vi "Vision Processor.vi"(5 "error in":errorcluster, 7 "Image In":T1) -> (0 "error out":errorcluster, 3 "Image Out":T1(plugin-control))   [LabVIEW 2013]
uses:
  <vilib>/vision/Image Controls.llb/IMAQ Image.ctl
  <vilib>/vision/NI_Vision_Development_Module.lvlib
panel:
  out "Cam":T1(plugin-control)
  # "0  center of mass x\n1  center of mass y\n2  first pixel x\n3  first pixel y\n4  bounding rect left\n5  bounding rect top\n6  bounding rect right\n7  bounding rect bottom\n8 max feret diameter start x\n9  max feret diameter start y\n10 max feret diameter end x\n11 max feret diameter end y\n12 max horiz segment length left\n13 max horiz segment length right\n14 max horiz segment length row\n15 bounding rect width \n16 bounding rect height\n17 bounding rect diagional\n..\n33 area"
  # "13'3\"\n3'9\""
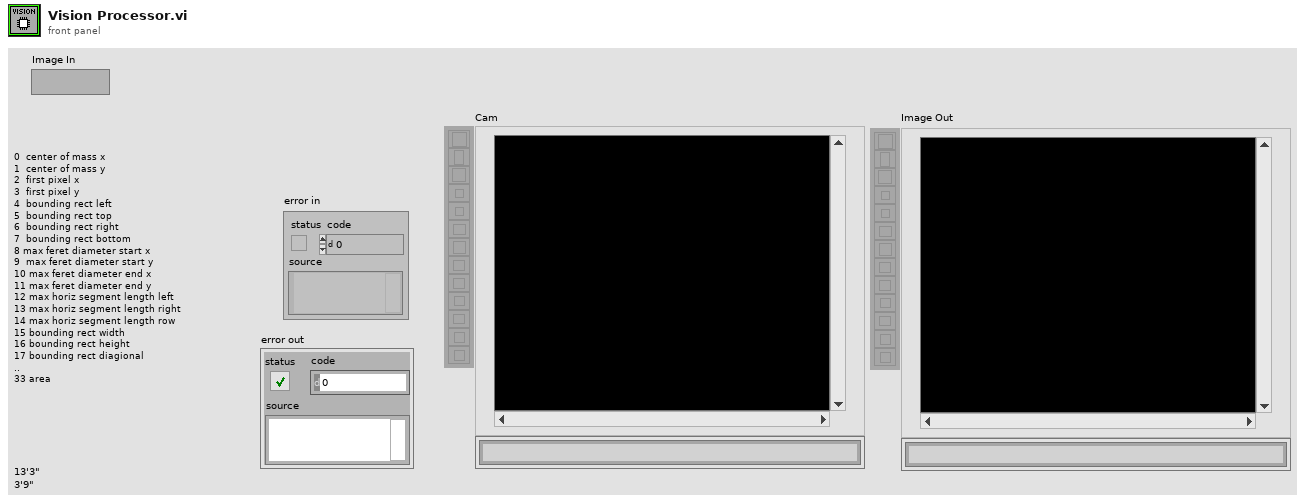
[diagram p1: front panel]
types:
  T1 = typedef "IMAQ Image.ctl" = refnum<image>
  T2 = enum32{"AutoM", "Close", "Dilate", "Erode", "Gradient", "Gradient out", "Gradient in", "Hit miss", "Open", "PClose", "POpen", "Thick", "Thin"}
  T3 = typedef "Image Type" = u32
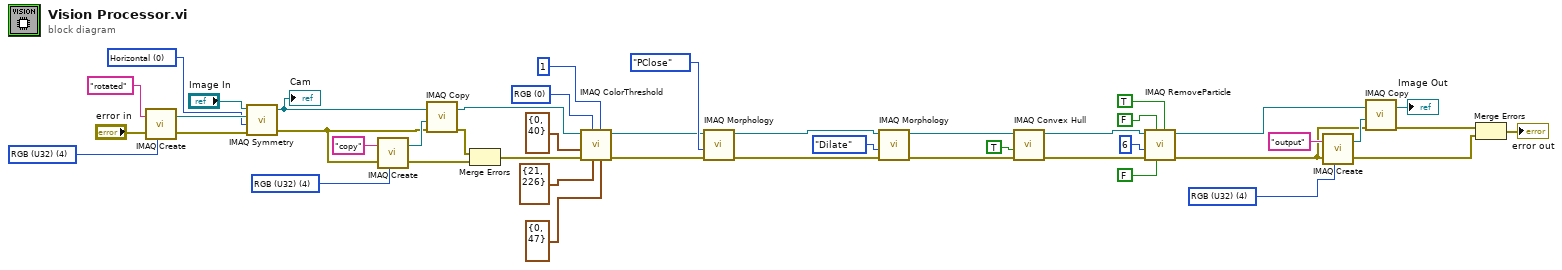
[diagram p0: block diagram]
diagram:
  w24 = T3 4 items=["Grayscale (U8)", "Grayscale (I16)", "Grayscale (SGL)", "Complex (CSG)", "RGB (U32)", "HSL (U32)", "RGB (U64)", "Grayscale (U16)"] ("Image Type")
  w30 = u32 0 items=["Horizontal", "Vertical", "Central", "1st Diagonal", "2nd Diagonal"] ("Type of Symmetry")
  w33 = T3 4 items=["Grayscale (U8)", "Grayscale (I16)", "Grayscale (SGL)", "Complex (CSG)", "RGB (U32)", "HSL (U32)", "RGB (U64)", "Grayscale (U16)"] ("Image Type")
  w35 = T3 4 items=["Grayscale (U8)", "Grayscale (I16)", "Grayscale (SGL)", "Complex (CSG)", "RGB (U32)", "HSL (U32)", "RGB (U64)", "Grayscale (U16)"] ("Image Type")
  w42 = u16 0 items=["RGB", "HSL", "HSV", "HSI"] ("Color Mode")
  n1 = call "IMAQ Create"("Image Name"="rotated", "Image Type"=w33, "error in (no error)"="error in") -> ("New Image"=w31:T1, "error out"=w8:errorcluster)  [unwired: 2 in]
  n2 = call "IMAQ Symmetry"("error in (no error)"=w8, "Type of Symmetry"=w30, "Image Dst"=w31, "Image Src"="Image In") -> ("error out"=w7:errorcluster, "Image Dst Out"=w14:T1)  [unwired: 1 in]
  "Cam" <- w14
  n3 = call "IMAQ Create"("Image Name"="copy", "Image Type"=w35, "error in (no error)"=w7) -> ("New Image"=w34:T1, "error out"=w6:errorcluster)  [unwired: 2 in]
  n4 = call "IMAQ Copy"("error in (no error)"=w7, "Image Dst"=w34, "Image Src"=w14) -> ("error out"=w5:errorcluster, "Image Dst Out"=w15:T1)  [unwired: 3 in]
  n5 = Merge Errors(w5, w6) -> (w4:errorcluster)
  n6 = call "IMAQ ColorThreshold"("Blue or Luma or Val or Inten Range"=cluster{"Lower value":i32, "Upper value":i32} {"Lower value"=0, "Upper value"=47}, "Replace Value"=1, "Green or Sat Range"=cluster{"Lower value":i32, "Upper value":i32} {"Lower value"=21, "Upper value"=226}, "Color Mode"=w42, "error in (no error)"=w4, "Red or Hue Range"=cluster{"Lower value":i32, "Upper value":i32} {"Lower value"=0, "Upper value"=40}, "Image Src"=w15) -> ("error out"=w27:errorcluster, "Image Dst Out"=w28:T1)  [unwired: 1 in, 2 out]
  n7 = call "IMAQ Morphology"("error in (no error)"=w27, "Operation"=T2."PClose", "Image Src"=w28) -> ("error out"=w19:errorcluster, "Image Dst Out"=w18:T1)  [unwired: 7 in]
  n8 = call "IMAQ Morphology"("error in (no error)"=w19, "Operation"=T2."Dilate", "Image Src"=w18) -> ("error out"=w16:errorcluster, "Image Dst Out"=w17:T1)  [unwired: 7 in]
  n9 = call "IMAQ Convex Hull"("error in (no error)"=w16, "Connectivity 4/8 (8)"=TRUE, "Image Src"=w17) -> ("error out"=w26:errorcluster, "Image Dst Out"=w25:T1)  [unwired: 1 in, 6 out]
  n10 = call "IMAQ RemoveParticle"("Connectivity 4/8 (8)"=TRUE, "Low Pass/High Pass (Low)"=FALSE, "Square/Hexa (Square)"=FALSE, "error in (no error)"=w26, "Number of Erosion"=6, "Image Src"=w25) -> ("error out"=w10:errorcluster, "Image Dst Out"=w21:T1)  [unwired: 1 in, 3 out]
  n11 = call "IMAQ Create"("Image Name"="output", "Image Type"=w24, "error in (no error)"=w10) -> ("New Image"=w22:T1, "error out"=w3:errorcluster)  [unwired: 2 in]
  n12 = call "IMAQ Copy"("error in (no error)"=w10, "Image Dst"=w22, "Image Src"=w21) -> ("error out"=w2:errorcluster, "Image Dst Out"=→"Image Out":T1)  [unwired: 3 in]
  n13 = Merge Errors(w2, w3) -> (→"error out":errorcluster)
